vi "getJoystickAxisForTankDrive.vi"(10 "Axes":dbl[](array[numeric]), 11 "Axes 2":dbl[](array[numeric])) -> (2 "Axes[0]":dbl, 3 "Axes[0] 2":dbl)   [LabVIEW 2014]
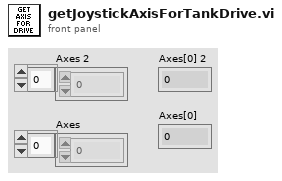
[diagram p1: front panel]
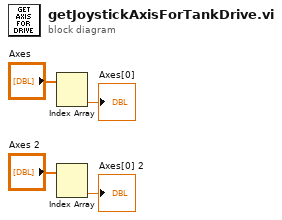
[diagram p0: block diagram]
diagram:
  n1 = Index Array(array="Axes") -> (element #2=→"Axes[0]":dbl)  [unwired: 2 in, 1 out]
  n2 = Index Array(array="Axes 2") -> (element #2=→"Axes[0] 2":dbl)  [unwired: 2 in, 1 out]
